vi "Abort Measurement.vi"(8 "error in":errorcluster, 11 "call ID in":T1) -> (0 "error out":errorcluster)   [LabVIEW 2025, in "Automotive Ethernet Bus Monitor_LabVIEW.lvlib"]
doc: "Cancel the ongoing measure call."
uses:
  Automotive Ethernet Bus Monitor_LabVIEW.lvlib
  <vilib>/gRPC/LabVIEW gRPC Library/Shared/grpcId.ctl
  <vilib>/gRPC/LabVIEW gRPC Library/grpc-lvsupport-release.lvlib
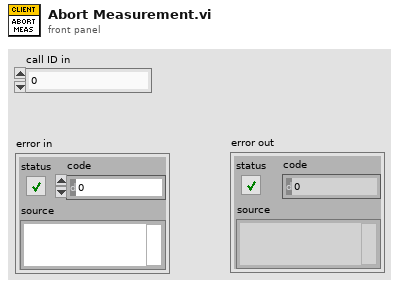
[diagram p1: front panel]
types:
  T1 = typedef "grpc-lvsupport-release.lvlib/grpcId.ctl" = u64
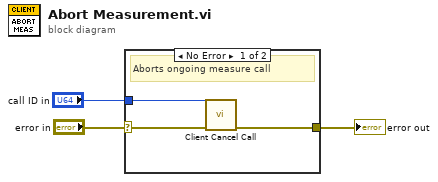
[diagram p0: block diagram]
diagram:
  n1 = case shown="No Error" "error in" {
    selector: "error in" -> [w6 w7]
    tunnel: [w5 w7] -> w2
    tunnel: "call ID in" -> [w4 _]
    frame No Error {
      # "Aborts ongoing measure call"
      n2 = call <vilib>:"Client Cancel Call.vi"("error in"=w6, "Call ID in"=w4) -> ("error out"=w5:errorcluster)  [unwired: 7 in, 2 out]
    }
    frame Error {
      # "Pass"
    }
  }
  "error out" <- w2
